vi "runs.get.vi"(8 "error in":errorcluster, 10 "rids":string[](array[string]), 11 "Nominal Client in":refnum<class "Nominal Client.lvclass">) -> (0 "error out":errorcluster, 2 "Runs":T1(array[cluster]), 3 "Nominal Client out":refnum<class "Nominal Client.lvclass">, 4 "Response body":string)   [LabVIEW 2020, in "Nominal Client.lvclass"]
uses:
  Nominal Client.lvclass
  49411445-db77-4211-b7bb-06afe579b778.vi
  e8484698-5fbf-4652-adfa-cc972abb1800.vi
  <vilib>/JDP Science/JSONtext/Variant to JSON Text.vi
  <vilib>/JDP Science/JSONtext/JSON text to Variant.vi
  <vilib>/JDP Science/JSONtext/LVClass Serializer/JSONtext LVClass Serializer.lvclass
  <vilib>/JDP Science/JSONtext/JSONtext.lvlib
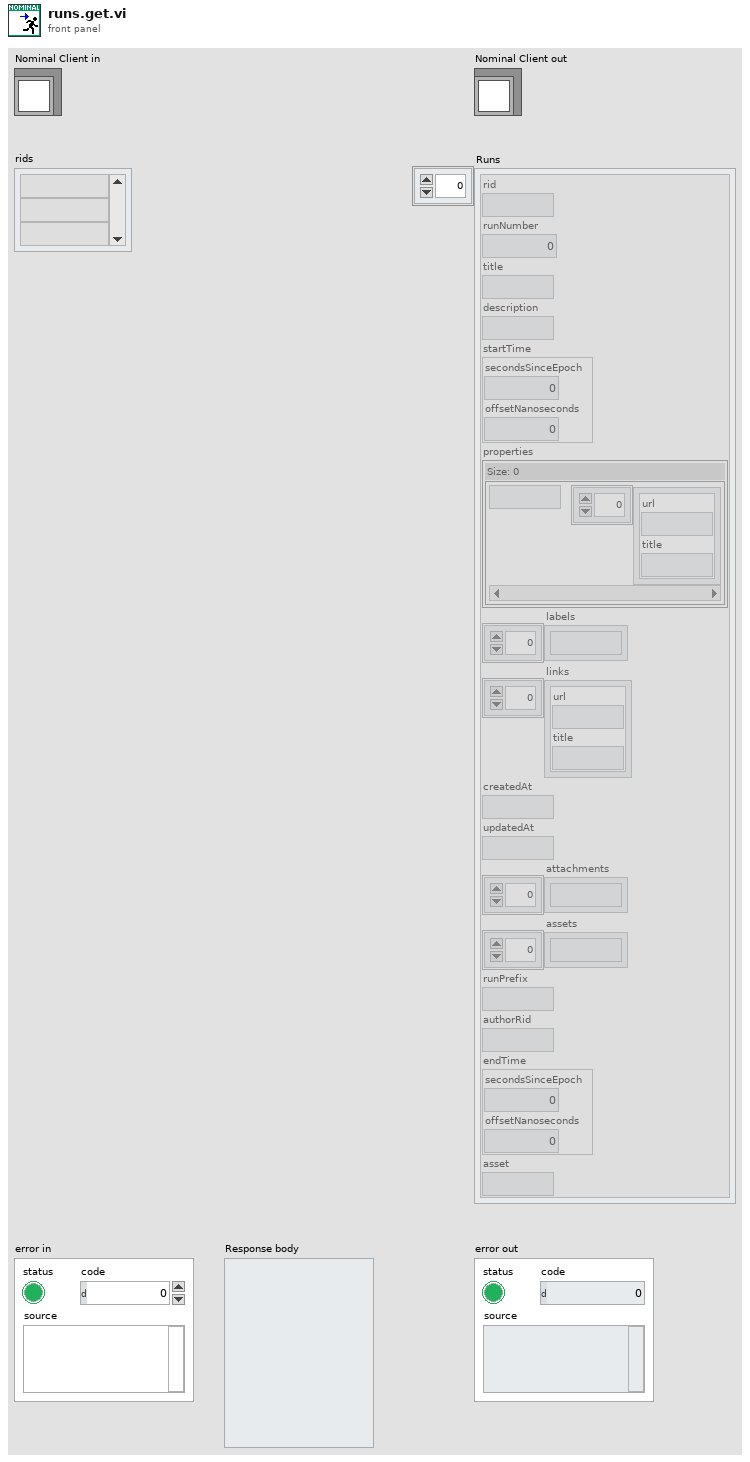
[diagram p1: front panel]
types:
  T1 = cluster{"rid":string, "runNumber":i32, "title":string, "description":string, "startTime":cluster{"secondsSinceEpoch":i32, "offsetNanoseconds":i32}, "properties":map{string, cluster{"url":string, "title":string}[]}, "labels":string[], "links":cluster{"url":string, "title":string}[], "createdAt":string, "updatedAt":string, "attachments":string[], "assets":string[], "runPrefix":string, "authorRid":string, "endTime":cluster{"secondsSinceEpoch":i32, "offsetNanoseconds":i32}, "asset":string}[]
  T2 = cluster{"rid":string, "runNumber":i32, "title":string, "description":string, "startTime":cluster{"secondsSinceEpoch":i32, "offsetNanoseconds":i32}, "properties":map{string, cluster{"url":string, "title":string}[]}, "labels":string[], "links":cluster{"url":string, "title":string}[], "createdAt":string, "updatedAt":string, "attachments":string[], "assets":string[], "runPrefix":string, "authorRid":string, "endTime":cluster{"secondsSinceEpoch":i32, "offsetNanoseconds":i32}, "asset":string}
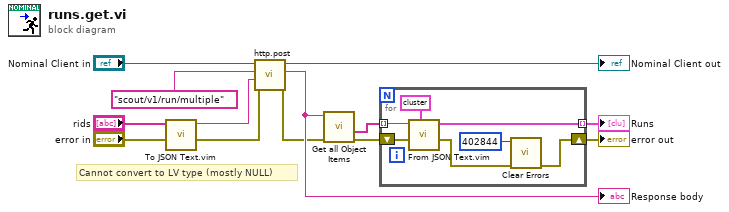
[diagram p0: block diagram]
diagram:
  # "Cannot convert to LV type (mostly NULL)"
  n1 = call "To JSON Text.vim"("error in (no error)"="error in", "Anything"="rids") -> ("error out"=w7:errorcluster, "<JSON>"=w9:string)  [unwired: 8 in]
  n2 = call "http.post.vi"("error in"=w7, "Request body"=w9, "Path"="scout/v1/run/multiple", "Nominal Client in"="Nominal Client in") -> ("error out"=w3:errorcluster, "Response"=w4:string, "Nominal Client out"=→"Nominal Client out":refnum<class "Nominal Client.lvclass">)  [unwired: 4 in, 1 out]
  "Response body" <- w4
  n3 = call <vilib>:"Get all Object Items.vi"("error in (no error)"=w3, "JSON"=w4) -> ("error out"=w5:errorcluster, "<JSON>"=w1:string[])  [unwired: 6 in, 2 out]
  n4 = for {
    tunnel: [w20] -> w6 mode=indexing
    shift-right: [w14] -> w2
    shift-left: w5 -> [w17]
    tunnel: w1 -> [w18] mode=indexing
    n5 = call "From JSON Text.vim"("Data Type and Default Value"=T2 {"rid"="", "runNumber"=0, "title"="", "description"="", "startTime"={"secondsSinceEpoch"=0, "offsetNanoseconds"=0}, "properties"={}, "labels"=[], "links"=[], "createdAt"="", "updatedAt"="", "attachments"=[], "assets"=[], "runPrefix"="", "authorRid"="", "endTime"={"secondsSinceEpoch"=0, "offsetNanoseconds"=0}, "asset"=""} ("Response"), "error in (no error)"=w17, "JSON"=w18) -> ("error out"=w15:errorcluster, "Data out"=w20:T2)  [unwired: 7 in]
    n6 = call <vilib>:"Clear Errors.vi"("error in (no error)"=w15, "specific error code to clear (0: all)"=402844) -> ("error out"=w14:errorcluster)  [unwired: 4 in, 1 out]
  }
  "error out" <- w2
  "Runs" <- w6
